vi "Initialize synthesizers.vi"(11 "VDI config constants in":T3={"Master"={"Lower limit [GHz]"=8.0, "Upper limit [GHz]"=20.0, "Name"="VDIS0122", "Handle"=0, "Description"="VDI Synth"}, "Follower"={"Lower limit [GHz]"=0.0, "Upper limit [GHz]"=20.0, "Name"="VDIYT7", "Handle"=0, "Description"="VDI Tracking"}}) -> (2 "Status":T1, 3 "VDI config constants out":T3={"Master"={"Lower limit [GHz]"=0.0, "Upper limit [GHz]"=0.0, "Name"="", "Handle"=0, "Description"=""}, "Follower"={"Lower limit [GHz]"=0.0, "Upper limit [GHz]"=20.0, "Name"="", "Handle"=0, "Description"=""}})   [LabVIEW 2021, in "THz source modeule.lvlib"]
uses:
  THz source modeule.lvlib
  ctl/VDI config constants.ctl
  ctl/Synth configs.ctl
  ctl/VDI status.ctl
  ctl/Synth status.ctl
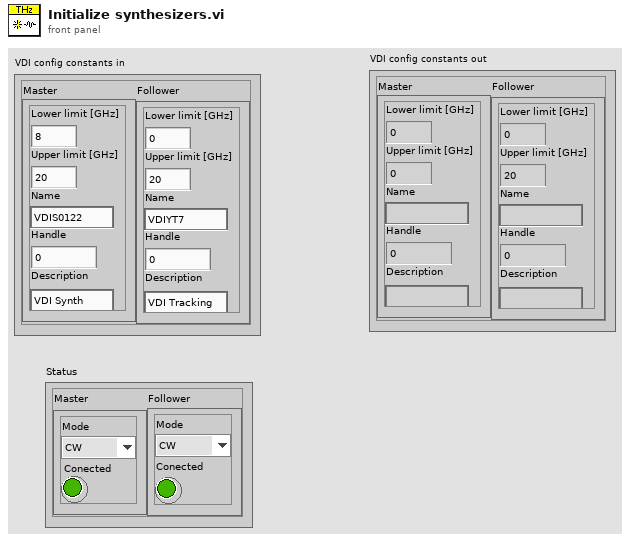
[diagram p1: front panel]
types:
  T1 = typedef "THz source modeule.lvlib/VDI status.ctl" = cluster{"Master":T2, "Follower":T2}
  T2 = typedef "THz source modeule.lvlib/Synth status.ctl" = cluster{"Mode":enum16{"CW", "Sweep"}, "Conected":bool}
  T3 = typedef "THz source modeule.lvlib/VDI config constants.ctl" = cluster{"Master":T4, "Follower":T4}
  T4 = typedef "THz source modeule.lvlib/Synth configs.ctl" = cluster{"Lower limit [GHz]":dbl, "Upper limit [GHz]":dbl, "Name":string, "Handle":u32, "Description":string}
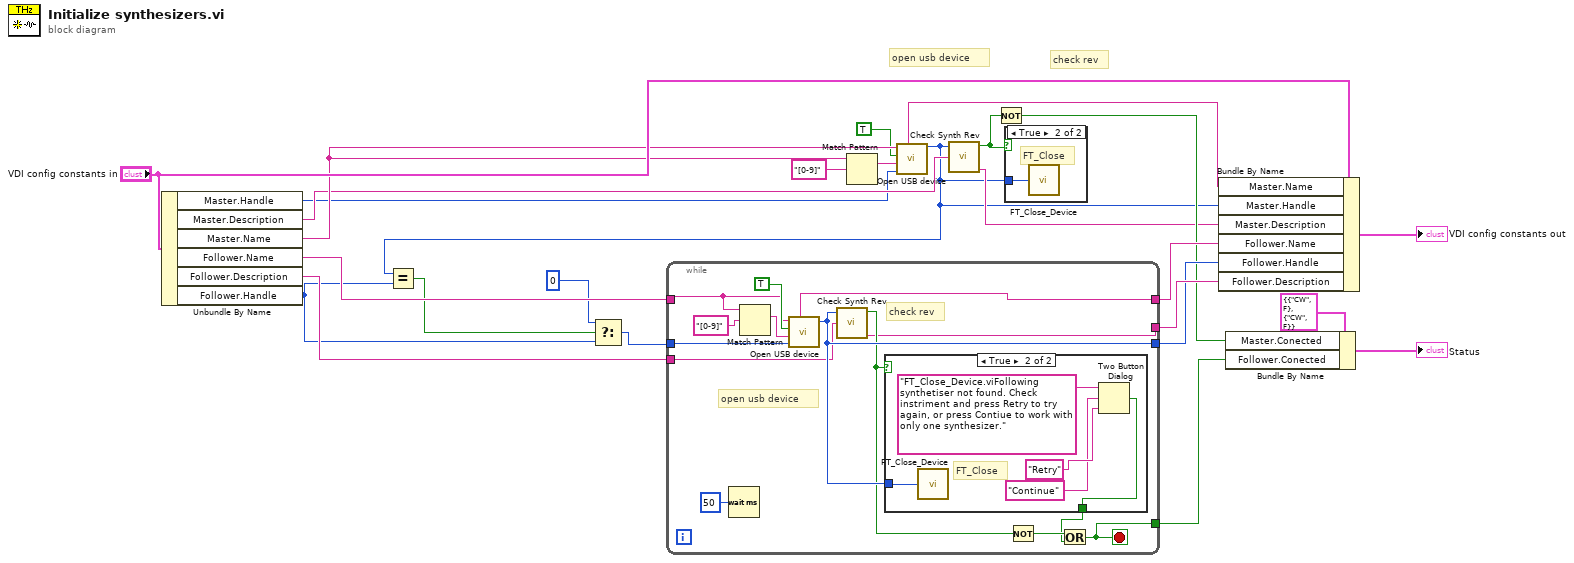
[diagram p0: block diagram]
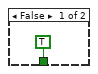
[diagram p2: hidden frame]
diagram:
  # "check rev"
  # "open usb device"
  n1 = Unbundle By Name("VDI config constants in") -> ("Master.Handle"=w2:u32, "Master.Description"=w10:string, "Master.Name"=w13:string, "Follower.Name"=w20:string, "Follower.Description"=w21:string, "Follower.Handle"=w6:u32)
  n2 = Match Pattern(string=w13, regular expression="[0-9]") -> (match substring=w12:string)  [unwired: 1 in, 3 out]
  n3 = call <instrlib>:"Open USB device.vi"("SN#"=w13, "close first"=TRUE, "Prefix"=w12, "Old handle"=w2) -> ("SN# out"=w11:string, "Handle out"=w1:u32)  [unwired: 2 out]
  n4 = Equal?(x=w1, y=w6) -> (x = y?=w7:bool)
  n5 = Select(t=u32 0, s=w7, f=w6) -> (s? t:f=w5:u32)
  n6 = while {
    tunnel: [w37] -> w25
    tunnel: w20 -> [w33]
    tunnel: [w30] -> w19
    tunnel: w21 -> [w27]
    tunnel: [w26] -> w24
    tunnel: w5 -> [w31]
    tunnel: [w29] -> w22
    stop <- w37 stop-if-true
    # "check rev"
    # "open usb device"
    n7 = Wait (ms)(milliseconds to wait=u32 50) -> ()  [unwired: 1 out]
    n8 = Match Pattern(string=w33, regular expression="[0-9]") -> (match substring=w32:string)  [unwired: 1 in, 3 out]
    n9 = call <instrlib>:"Open USB device.vi"("SN#"=w33, "close first"=TRUE, "Prefix"=w32, "Old handle"=w31) -> ("SN# out"=w30:string, "Handle out"=w29:u32)  [unwired: 2 out]
    n10 = call <instrlib>:"Check Synth Rev.vi"("Handle"=w29, "Description"=w27) -> ("Wrong Rev"=w28:bool, "Device Description"=w26:string)  [unwired: 7 in]
    n11 = case shown="True" w28 {
      tunnel: w29 -> [_ w41]
      tunnel: [TRUE ("T button?") w44] -> w36
      frame False {
      }
      frame True {
        # "FT_Close"
        n12 = call <instrlib>:"FT_Close_Device.vi"("Handle"=w41) -> ()  [unwired: 1 out]
        n13 = Two Button Dialog(message="FT_Close_Device.viFollowing synthetiser not found. Check instriment and press Retry to try again, or press Contiue to work with only one synthesizer.", 1:"Retry" ("T button name (\"OK\")"), 2:"Continue" ("F button name (\"Cancel\")")) -> (T button?=w44:bool)
      }
    }
    n14 = Not(x=w28) -> (.not. x?=w38:bool)
    n15 = Or(x=w38, y=w36) -> (x .or. y?=w37:bool)
  }
  n16 = call <instrlib>:"Check Synth Rev.vi"("Handle"=w1, "Description"=w10) -> ("Wrong Rev"=w4:bool, "Device Description"=w8:string)  [unwired: 7 in]
  n17 = Not(x=w4) -> (.not. x?=w14:bool)
  n18 = case shown="True" w4 {
    tunnel: w1 -> [_ w46]
    frame False {
    }
    frame True {
      # "FT_Close"
      n19 = call <instrlib>:"FT_Close_Device.vi"("Handle"=w46) -> ()  [unwired: 1 out]
    }
  }
  n20 = Bundle By Name(cluster="VDI config constants in", "Master.Name"=w11, "Master.Handle"=w1, "Master.Description"=w8, "Follower.Name"=w19, "Follower.Handle"=w22, "Follower.Description"=w24) -> (→"VDI config constants out":T3)
  n21 = Bundle By Name(cluster=T1 {"Master"={"Mode"=enum."CW", "Conected"=FALSE}, "Follower"={"Mode"=enum."CW", "Conected"=FALSE}}, "Master.Conected"=w14, "Follower.Conected"=w25) -> (→"Status":T1)
